vi "loadProjectWithMacro.vi"(8 "error in (no error)":errorcluster, 9 "macro":string, 10 "projectName":string, 11 "VGS_RemoteControlClient in":refnum<class "VGS_RemoteControlClient.lvclass">) -> (0 "error out":errorcluster, 3 "VGS_RemoteControlClient out":refnum<class "VGS_RemoteControlClient.lvclass">)   [LabVIEW 2022 SP3, in "LV_VGS.lvlib" / "VGS_RemoteControlClient.lvclass"]
doc: "<B>Loads a VG project into an existing VGStudio MAX instance and play a macro. </B>\n\nThis method loads the specified VG project into a VGStudio (MAX) instance. Thereafter the macro will be played on the loaded VG project. The absolute path name to the VG project and macro file will be passed.\n\nThe remote controlled application must be VGStudio MAX 2.1 and higher. The remote computer on which VGStudio MAX is running must be able to read this VG project. \n\nParameters\nhandle A valid remote handle. \nprojectName The absolute path to the VG project. \nmacro The absolute path to a VG macro file (.vgc) is passed. \n\nEmit error ApplicationHasNoMacroSupportException if the current application instance has no macro support e.g. VGStudio or myVGL. \nEmit error RemoteControlServiceIsNotAvailableException if the remote control service doesn't run. \nEmit error GenericRemoteControlErrorException if an internal error occurs.\nEmit error InvalidRemoteHandleException if the remote handle is not valid."
uses:
  VGS_RemoteControlClient.lvclass
  VGS_RemoteControlClient.lvclass/VGS_RemoteControlClient.ctl
  C:/Users/Andrey/Documents/GitHub/LV_VGS/vgs_project.dll
  vgs_project.dll
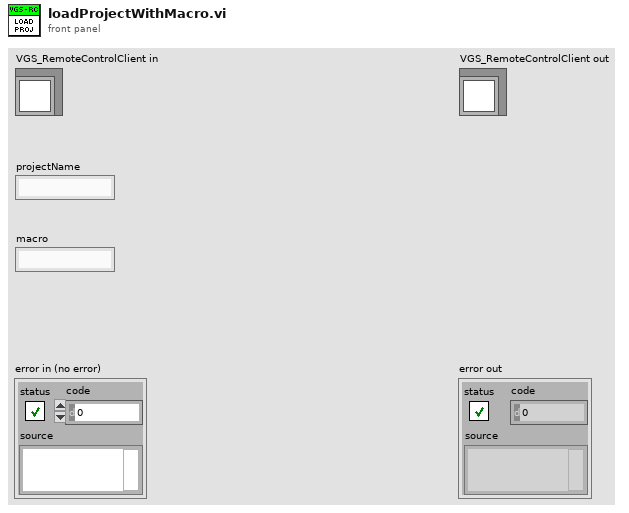
[diagram p1: front panel]
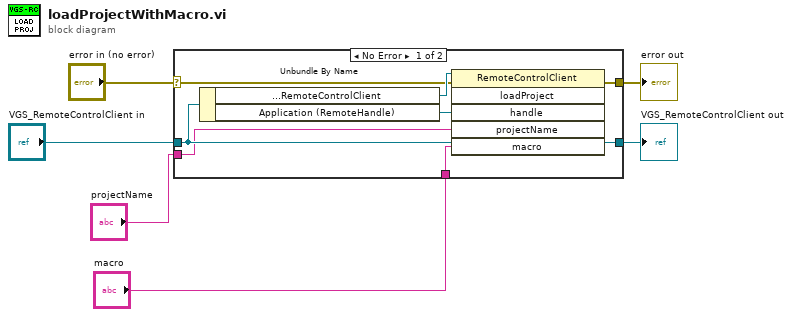
[diagram p0: block diagram]
diagram:
  n1 = case shown="No Error" "error in (no error)" {
    selector: "error in (no error)" -> [w9 w14]
    tunnel: [w8 w14] -> w5
    tunnel: [w13 w15] -> w3
    tunnel: "VGS_RemoteControlClient in" -> [w13 w15]
    tunnel: "projectName" -> [w10 _]
    tunnel: "macro" -> [w7 _]
    frame No Error {
      n2 = Unbundle By Name(w13) -> ("VGS.Project.Interop.RemoteControlClient"=w12:refnum<k24>, "Application (RemoteHandle)"=w11:refnum<k24>)
      n3 = invoke class="RemoteControlClient" method="loadProject"(reference=w12, error in=w9, "handle"=w11, "projectName"=w10, "macro"=w7) -> (error out=w8:errorcluster)  [unwired: 1 in, 5 out]
    }
    frame Error {
    }
  }
  "error out" <- w5
  "VGS_RemoteControlClient out" <- w3
